vi "Centrifuge Out Selection.vi"(8 "error in (no error)":errorcluster, 10 "Speed":dbl, 11 "Pump Settings In":T1={"Output Device"=enum."Default", "EPOS4 Settings"={"VISA resource name"="", "axis"={"keyHandle"=1, "nodeId"=1}, "Simulated?"=FALSE}}) -> (0 "error out":errorcluster, 2 "Connection Error":bool, 3 "Pump Settings Out":T1={"Output Device"=enum."Default", "EPOS4 Settings"={"VISA resource name"="", "axis"={"keyHandle"=1, "nodeId"=1}, "Simulated?"=FALSE}})   [LabVIEW 2018, in "Centrifuge Module.lvlib" / "Centrifuge Module Engine.lvlib"]
uses:
  Centrifuge Module Engine.lvlib
  Centrifuge Settings Cluster.ctl
  EPOS4/Controls/Device Selection.ctl
  EPOS4/Controls/EPOS Communication Settings.ctl
  Centrifuge Module.lvlib
  EPOS4/EPOS4.lvlib
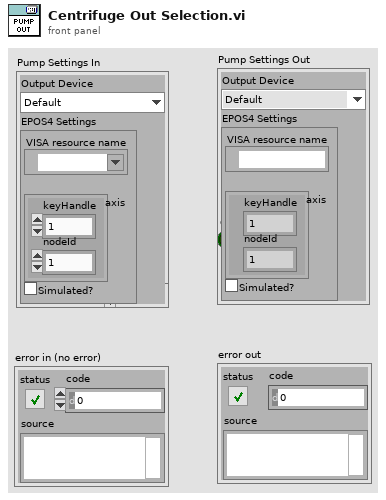
[diagram p1: front panel]
types:
  T1 = typedef "Centrifuge Module.lvlib/Centrifuge Settings Cluster.ctl" = cluster{"Output Device":T2, "EPOS4 Settings":T3}
  T2 = typedef "Device Selection.ctl" = enum16{"Default", "EPOS4"}
  T3 = typedef "EPOS4.lvlib/EPOS Communication Settings.ctl" = cluster{"VISA resource name":refnum<visa-resource-name>, "axis":cluster{"keyHandle":u32, "nodeId":u16}, "Simulated?":bool}
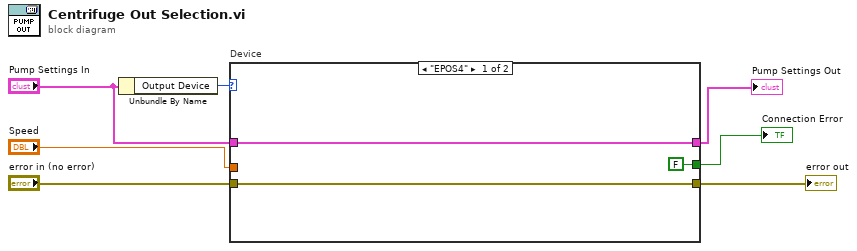
[diagram p0: block diagram]
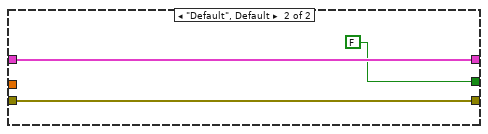
[diagram p2: hidden frame]
diagram:
  n1 = Unbundle By Name("Pump Settings In") -> ("Output Device"=w3:T2)
  n2 = case "Device" shown="\"EPOS4\"" w3 {
    tunnel: "Speed" -> [_ _]
    tunnel: "error in (no error)" -> [w10 w12]
    tunnel: [w10 w12] -> w6
    tunnel: "Pump Settings In" -> [w9 w13]
    tunnel: [w9 w13] -> w2
    tunnel: [FALSE ("Connection Error") FALSE ("Connection Error")] -> w7
    frame "EPOS4" {
    }
    frame "Default", Default {
    }
  }
  "Connection Error" <- w7
  "error out" <- w6
  "Pump Settings Out" <- w2
